vi "set_maximum_output_value.vi"(8 "error in (no error)":errorcluster, 10 "maximum output value":dbl, 11 "DAQmxWriteSignals.lvclass in":refnum<class "SignalWriterMM140725DAQmx.lvclass">) -> (0 "error out":errorcluster, 3 "DAQmxWriteSignals.lvclass out":refnum<class "SignalWriterMM140725DAQmx.lvclass">)   [LabVIEW 2010, in "SignalWriterMM140725DAQmx.lvclass"]
uses:
  SignalWriterMM140725DAQmx.lvclass
  GenericSignalWriter/GenericSignalWriter/GenericSignalWriter.lvclass
  SignalWriterMM140725DAQmx.lvclass/SignalWriterMM140725DAQmx.ctl
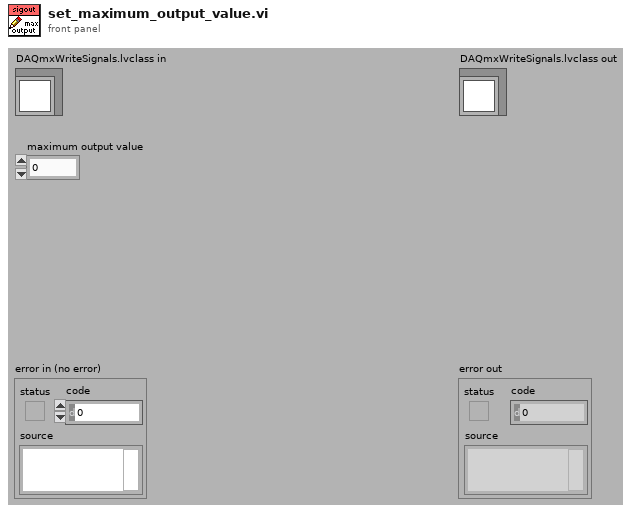
[diagram p1: front panel]
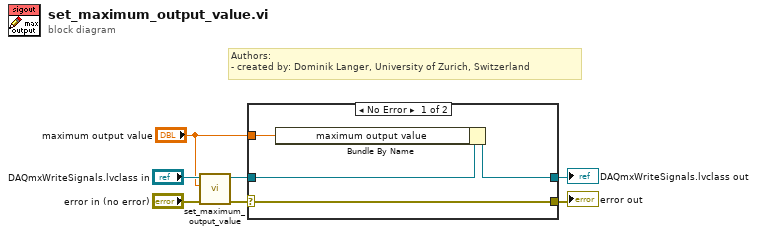
[diagram p0: block diagram]
diagram:
  # "Authors: \n- created by: Dominik Langer, University of Zurich, Switzerland"
  n1 = call-parent "set_maximum_output_value.vi"("error in (no error)"="error in (no error)", "maximum output value"="maximum output value", "GenericWriteSignals.lvclass in"="DAQmxWriteSignals.lvclass in") -> ("error out"=w5:errorcluster, "GenericWriteSignals.lvclass out"=w4:refnum<class "SignalWriterMM140725DAQmx.lvclass">)  [unwired: 7 out]
  n2 = case shown="No Error" w5 {
    selector: w5 -> [w8 w13]
    tunnel: w4 -> [w11 w12]
    tunnel: [w8 w13] -> w3
    tunnel: [w9 w12] -> w2
    tunnel: "maximum output value" -> [w10 _]
    frame No Error {
      n3 = Bundle By Name(cluster=w11, "maximum output value"=w10) -> (w9:refnum<class "SignalWriterMM140725DAQmx.lvclass">)
    }
    frame Error {
    }
  }
  "error out" <- w3
  "DAQmxWriteSignals.lvclass out" <- w2
